vi "instrumentProperties_PDTemperatureMode_available.vi"(0 "reference":refnum<class "OSA300.lvclass">, 5 "error in (no error)":errorcluster) -> (14 "duplicate reference":refnum<class "OSA300.lvclass">, 16 "PDTempCtrl_available":bool, 19 "error out":errorcluster)   [LabVIEW 2010, in "OSA300.lvclass"]
doc: "Returns boolean true if the active channel photodetector, (channel assigned for acquisition), is held at constant low temperature, (cooled).\n\nNote - OSA200 series has only one channel."
uses:
  OSA300.lvclass
  OSA300.lvclass/OSA300.ctl
  _OSAchannel_class/OSAchannel.lvclass
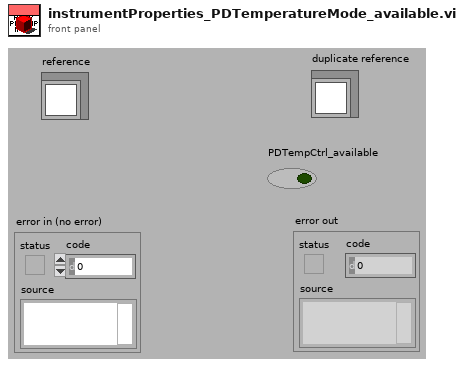
[diagram p1: front panel]
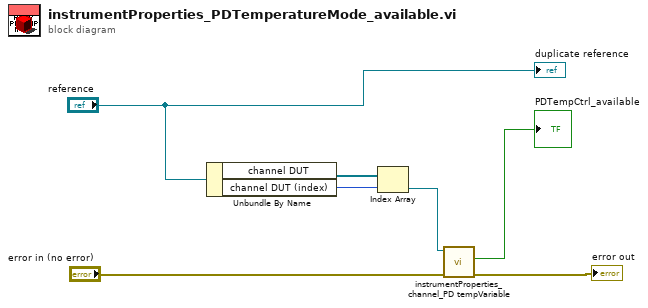
[diagram p0: block diagram]
diagram:
  n1 = Unbundle By Name("reference") -> ("channel DUT"=w7:refnum<class "OSAchannel.lvclass">[], "channel DUT (index)"=w6:i32)
  n2 = Index Array(array=w7, index=w6) -> (element=w5:refnum<class "OSAchannel.lvclass">)
  n3 = call "instrumentProperties_channel_PD tempVariable.vi"("error in (no error)"="error in (no error)", "OSAchannel in"=w5) -> ("error out"=→"error out":errorcluster, "tempVar_available"=→"PDTempCtrl_available":bool)  [unwired: 7 in, 1 out]
  "duplicate reference" <- "reference"
